vi "SlewRateLimiter_NewInitialZero.vi"(11 "RateLimit":dbl) -> (3 "out SLEW_RATE_LIMITER":T1 {"PrevTime" format="%30.5p"; "PrevValue" format="%13.5p"; "RateLimit" format="%13.5p"})   [LabVIEW 2019, in "Trajectory_Library.lvlib"]
doc: "Creates a new SlewRateLimiter data cluster with the given rate limit. The initial value is set to zero.\n\nThis set of functions limits the rate of change of an input value. Useful for implementing voltage, setpoint, and/or output ramps. A slew-rate limit is most appropriate when the quantity being controlled is a velocity or a voltage; when controlling a position, consider using a postion control algoritmn or trapezoid profile instead.\n\nInputs:\n - rateLimit -- The rate-of-change limit, in units per second.\n \nOutputs:\n - out Slew Rate Limiter -- The initialized Slew Rate Limiter data cluster"
uses:
  Trajectory_Library.lvlib
  SLEW_RATE_LIMITER.ctl
  Util_GetTime.vi
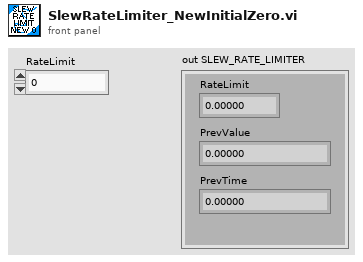
[diagram p1: front panel]
types:
  T1 = typedef "Trajectory_Library.lvlib/SLEW_RATE_LIMITER.ctl" = cluster{"RateLimit":dbl, "PrevValue":dbl, "PrevTime":dbl}
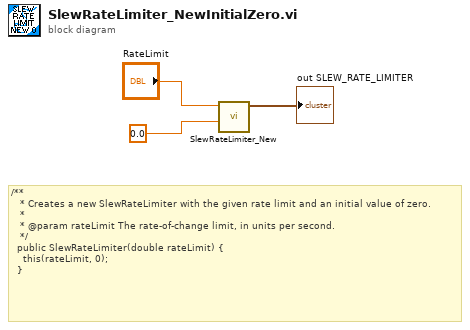
[diagram p0: block diagram]
diagram:
  # "/**\n   * Creates a new SlewRateLimiter with the given rate limit and an initial value of zero.\n   *\n   * @param rateLimit The rate-of-change limit, in units per second.\n   */\n  public SlewRateLimiter(double rateLimit) {\n    this(rateLimit, 0);\n  }"
  n1 = call "SlewRateLimiter_New.vi"("InitialValue"=0.0, "RateLimit"="RateLimit") -> ("out SLEW_RATE_LIMITER"=→"out SLEW_RATE_LIMITER":T1)  [unwired: 9 in]
